vi "Lower Front Arms.vi"(11 "Button":bool) -> ()   [LabVIEW 2014]
uses:
  Robot Global Data.vi
  Desired Arm Position.vi
panel:
  in  "desired drop":dbl=10.0
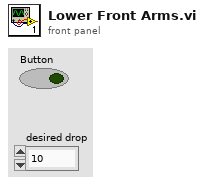
[diagram p1: front panel]
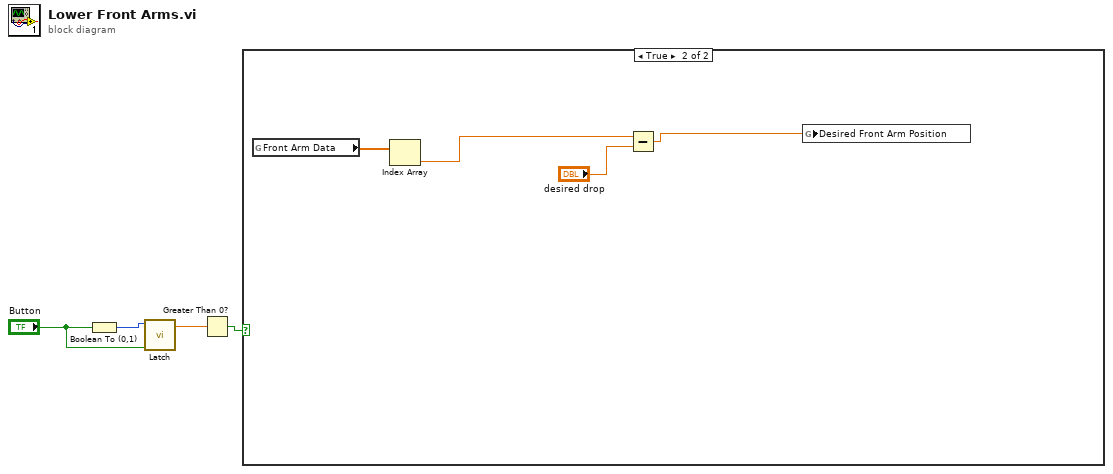
[diagram p0: block diagram]
diagram:
  n1 = Boolean To (0,1)(Boolean="Button") -> (0, 1=w4:i16)
  n2 = call "Latch.vi"("Reset"="Button", "Input"=w4) -> ("Output"=w2:dbl)  [unwired: 9 in]
  n3 = Greater Than 0?(x=w2) -> (x > 0?=w3:bool)
  n4 = case shown="True" w3 {
    frame False {
    }
    frame True {
      n5 = global read "Robot Global Data.vi" "Front Arm Data"() -> (w6:dbl[])
      n6 = Index Array(array=w6) -> (element=w5:dbl)  [unwired: 1 in]
      n7 = Subtract(x=w5, y="desired drop") -> (x-y=w8:dbl)
      n8 = global write "Desired Arm Position.vi" "Desired Front Arm Position"(w8) -> ()
    }
  }
